vi "Listen.vi"(8 "error in (no error)":errorcluster caption="错误输入（无错误）", 11 "MainPage 输入":refnum<class "MainPage.lvclass">) -> (0 "error out":errorcluster caption="错误输出", 3 "MainPage 输出":refnum<class "MainPage.lvclass">)   [LabVIEW 2019, in "MainPage.lvlib" / "MainPage.lvclass"]
uses:
  MainPage.lvclass
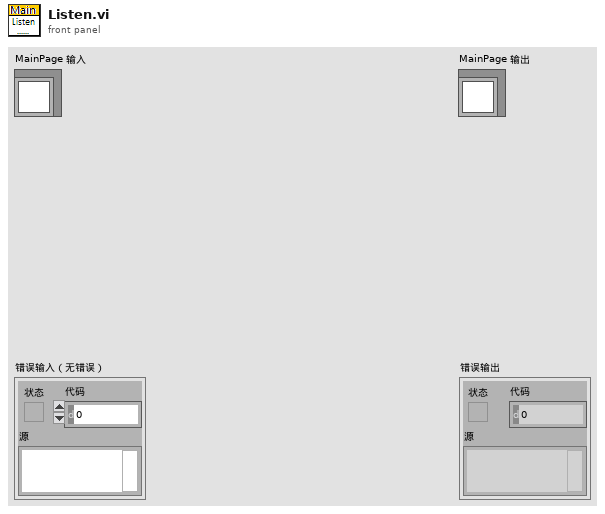
[diagram p1: front panel]
types:
  T1 = enum16{"Standard", "Buffered", "CRLF", "Immediate"}
  T2 = typedef "MainPage.lvlib/MainPage.lvclass/DataRef_通讯接口.ctl" = cluster{"连接方式":enum16{"网口(客服端)", "网口(服务端)", "串口"}, "VISA串口名称":refnum<visa-resource-name>, "服务端识别":cluster{"本机IP":string, "本机端口":u16, "当前目标":string}, "客服端识别":cluster{"当前端口":u16, "目标IP":string, "目标端口":u16}, "服务端记录":cluster{"服务端侦听ID":refnum<k5>, "服务端接口记录":map{string, cluster{"连接ID":refnum<k5>}}}, "客服端记录":map{u16, cluster{"连接ID":refnum<k5>}}, "侦听周期(ms)":u32}
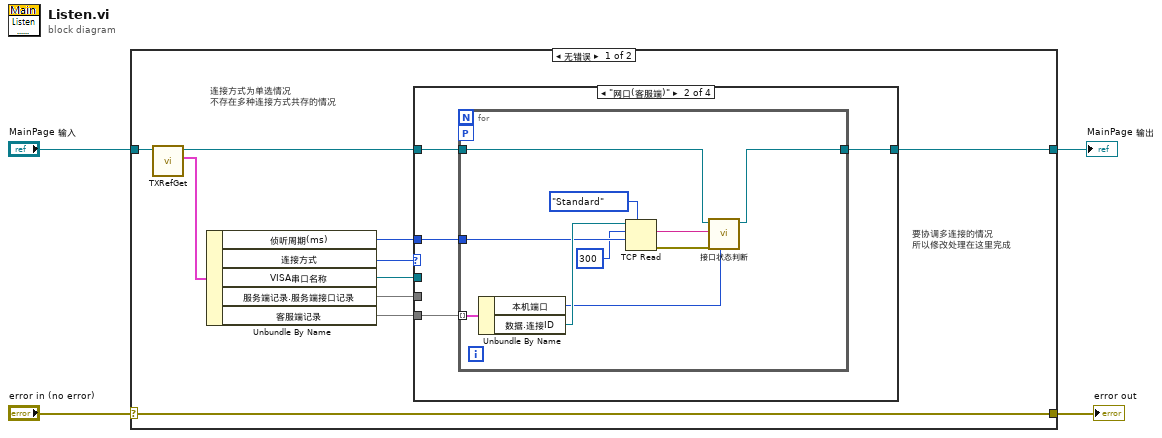
[diagram p0: block diagram]
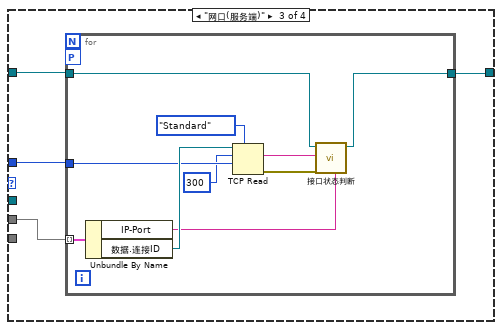
[diagram p3: hidden frame]
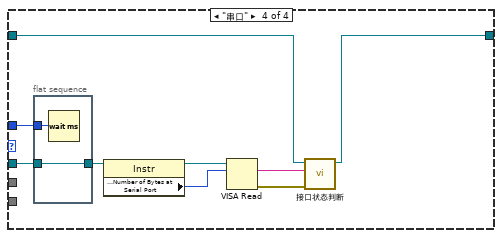
[diagram p4: hidden frame]
diagram:
  n1 = case shown="无错误" "error in (no error)" {
    selector: "error in (no error)" -> [w14 w56]
    tunnel: [w14 w56] -> w3
    tunnel: [w7 w55] -> w1
    tunnel: "MainPage 输入" -> [w13 w55]
    frame No Error {
      # "要协调多连接的情况\n所以修改处理在这里完成"
      # "连接方式为单选情况\n不存在多种连接方式共存的情况"
      n2 = call-dynamic "TXRefGet.vi"("MainPage 输入"=w13) -> ("通讯接口数据"=w12:T2, "MainPage 输出"=w8:refnum<class "MainPage.lvclass">)  [unwired: 6 in, 3 out]
      n3 = Unbundle By Name(w12) -> ("侦听周期(ms)"=w9:u32, "连接方式"=w11:enum16{"网口(客服端)", "网口(服务端)", "串口"}, "VISA串口名称"=w10:refnum<visa-resource-name>, "服务端记录.服务端接口记录"=w6:map{string, cluster{"连接ID":refnum<k5>}}, "客服端记录"=w5:map{u16, cluster{"连接ID":refnum<k5>}})
      n4 = case shown="\"网口(客服端)\"" w11 {
        tunnel: w10 -> [_ _ _ w49]
        tunnel: w9 -> [_ w16 w30 w50]
        tunnel: w8 -> [w15 w19 w33 w45]
        tunnel: [w15 w18 w32 w46] -> w7
        tunnel: w6 -> [_ _ w31 _]
        tunnel: w5 -> [_ w17 _ _]
        frame Default {
        }
        frame "网口(客服端)" {
          n5 = for {
            workers-P: _ -> [_]
            tunnel: w19 -> [w25]
            tunnel: [w24] -> w18
            tunnel: w17 -> [w29] mode=indexing
            tunnel: w16 -> [w27]
            n6 = Unbundle By Name(w29) -> ("本机端口"=w22:u16, "数据.连接ID"=w28:refnum<k5>)
            n7 = TCP Read(connection ID=w28, bytes to read=300 ("读取的字节"), 7:T1."Standard" ("模式（标准）"), 9:w27) -> (data out=w20:string, error out=w23:errorcluster)  [unwired: 1 in, 1 out]
            n8 = call "接口状态判断.vi"("本机端口"=w22, "error in (no error)"=w23, "报文"=w20, "MainPage 输入"=w25) -> ("MainPage 输出"=w24:refnum<class "MainPage.lvclass">)  [unwired: 6 in, 1 out]
          }
        }
        frame "网口(服务端)" {
          n9 = for {
            workers-P: _ -> [_]
            tunnel: w33 -> [w39]
            tunnel: [w38] -> w32
            tunnel: w31 -> [w43] mode=indexing
            tunnel: w30 -> [w41]
            n10 = Unbundle By Name(w43) -> ("IP-Port"=w35:string, "数据.连接ID"=w42:refnum<k5>)
            n11 = TCP Read(connection ID=w42, bytes to read=300 ("读取的字节"), 7:T1."Standard" ("模式（标准）"), 9:w41) -> (data out=w34:string, error out=w37:errorcluster)  [unwired: 1 in, 1 out]
            n12 = call "接口状态判断.vi"("IP-Port"=w35, "error in (no error)"=w37, "报文"=w34, "MainPage 输入"=w39) -> ("MainPage 输出"=w38:refnum<class "MainPage.lvclass">)  [unwired: 6 in, 1 out]
          }
        }
        frame "串口" {
          n13 = flat-sequence {
            tunnel: w50 -> [w54]
            tunnel: w49 -> [w53]
            tunnel: [w53] -> w48
            frame #0 {
              n14 = Wait (ms)(milliseconds to wait=w54) -> ()  [unwired: 1 out]
            }
          }
          n15 = property class="Instr"(reference=w48) -> (reference out=w52:refnum<visa-resource-name>, "Serial Settings:Number of Bytes at Serial Port"=w51:u32)  [unwired: 1 in, 1 out]
          n16 = VISA Read(VISA resource name=w52, byte count=w51) -> (read buffer=w44:string, error out=w47:errorcluster)  [unwired: 1 in, 2 out]
          n17 = call "接口状态判断.vi"("error in (no error)"=w47, "报文"=w44, "MainPage 输入"=w45) -> ("MainPage 输出"=w46:refnum<class "MainPage.lvclass">)  [unwired: 7 in, 1 out]
        }
      }
    }
    frame Error {
    }
  }
  "error out" <- w3
  "MainPage 输出" <- w1
